vi "Get Executable Attributes.vi"(8 "error in (no error)":errorcluster, 11 "WriteCommand in":refnum<class "WriteCommand.lvclass">) -> (0 "error out":errorcluster, 2 "Executable Attributes":T1, 3 "WriteCommand out":refnum<class "WriteCommand.lvclass">)   [LabVIEW 2023, in "HAF.lvlib" / "WriteCommand.lvclass"]
doc: "Provides a set of attributes that are used to control how the Driver should run the Executable on an Instrument."
uses:
  WriteCommand.lvclass
  WriteCommand.lvclass/WriteCommand.ctl
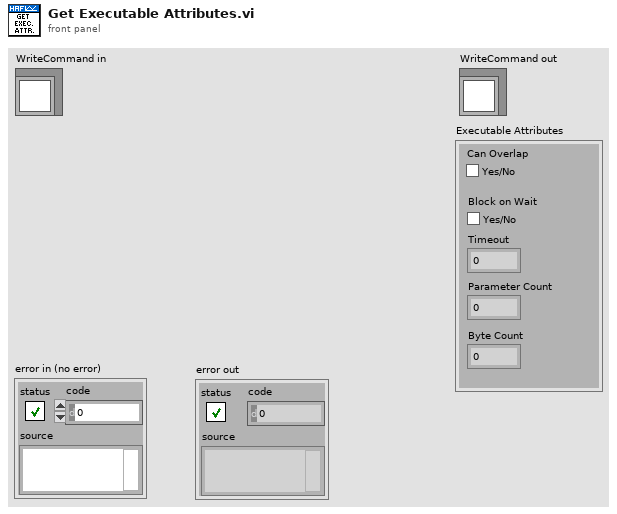
[diagram p1: front panel]
types:
  T1 = cluster{"Can Overlap":bool, "Block on Wait":bool, "Timeout":u32, "Byte Count":u32, "Parameter Count":u32}
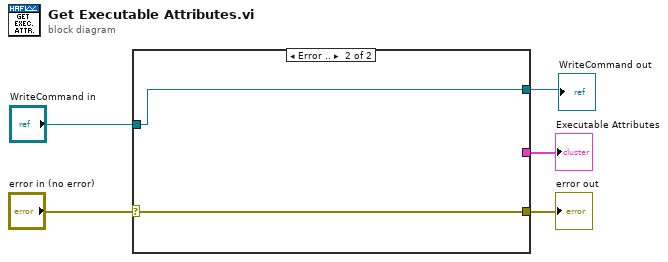
[diagram p0: block diagram]
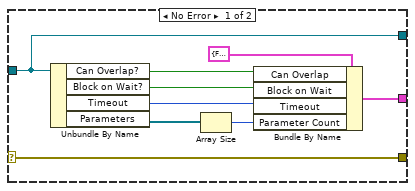
[diagram p2: hidden frame]
diagram:
  n1 = case shown="Error .." "error in (no error)" {
    selector: "error in (no error)" -> [w14 w15]
    tunnel: "WriteCommand in" -> [w13 w16]
    tunnel: [w14 w15] -> w3
    tunnel: [w13 w16] -> w2
    tunnel: [w6 _] -> w1
    frame No Error {
      n2 = Unbundle By Name(w13) -> ("Can Overlap?"=w11:bool, "Block on Wait?"=w10:bool, "Timeout"=w9:u32, "Parameters"=w7:refnum<class "Parameter.lvclass">[])
      n3 = Array Size(array=w7) -> (size(s)=w8:i32)
      n4 = Bundle By Name(cluster=T1 {"Can Overlap"=FALSE, "Block on Wait"=FALSE, "Timeout"=0, "Byte Count"=0, "Parameter Count"=0} ("Executable Attributes"), "Can Overlap"=w11, "Block on Wait"=w10, "Timeout"=w9, "Parameter Count"=w8) -> (w6:T1)
    }
    frame Error {
    }
  }
  "error out" <- w3
  "WriteCommand out" <- w2
  "Executable Attributes" <- w1
